vi "Array Template.vi"   [LabVIEW 2012]
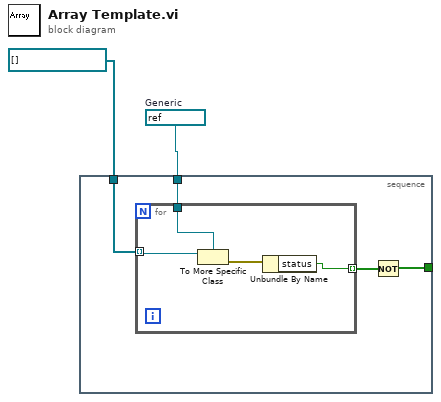
[diagram p0: block diagram]
diagram:
  w2 = refnum<vi> refnum  # Generic
  n1 = stacked-sequence {
    tunnel: [w3] -> _
    tunnel: w2 -> [w5]
    tunnel: refnum<vi>[] [] -> [w4]
    frame #0 {
      n2 = for {
        tunnel: [w9] -> w6 mode=indexing
        tunnel: w5 -> [w8]
        tunnel: w4 -> [w7] mode=indexing
        n3 = To More Specific Class(target class=w8, reference=w7) -> (error out=w10:errorcluster)  [unwired: 1 in, 1 out]
        n4 = Unbundle By Name(w10) -> ("status"=w9:bool)
      }
      n5 = Not(x=w6) -> (.not. x?=w3:bool[])
    }
  }
